vi "approach.vi"(8 "error in (no error)":errorcluster, 11 "Input":string="f") -> (0 "error out":errorcluster, 3 "Output":string="approached")   [LabVIEW 2014]
uses:
  <userlib>/Nanonis Prog Interface V5/Nanonis Prog Interface.lvlib
  <userlib>/SSL Library/SSL Lib.lvlib
panel:
  in  "Amplitude (V) (NaN=no change)":sgl=200.0
  in  "Frequency (Hz) (NaN=no change)":sgl=1000.0
  out "testing?":bool
  in  "STMStatus":T1 {"Size (m)"."Height" format="%.2p"; "Size (m)"."Width" format="%.2p"; "Current (A)" format="%#_6p"; "Z position (m)" format="%#_6p"; "Center coordinates (m)"."Yc" format="%.2p"; "Center coordinates (m)"."Xc" format="%.2p"}
  out "size(s)":i32=1
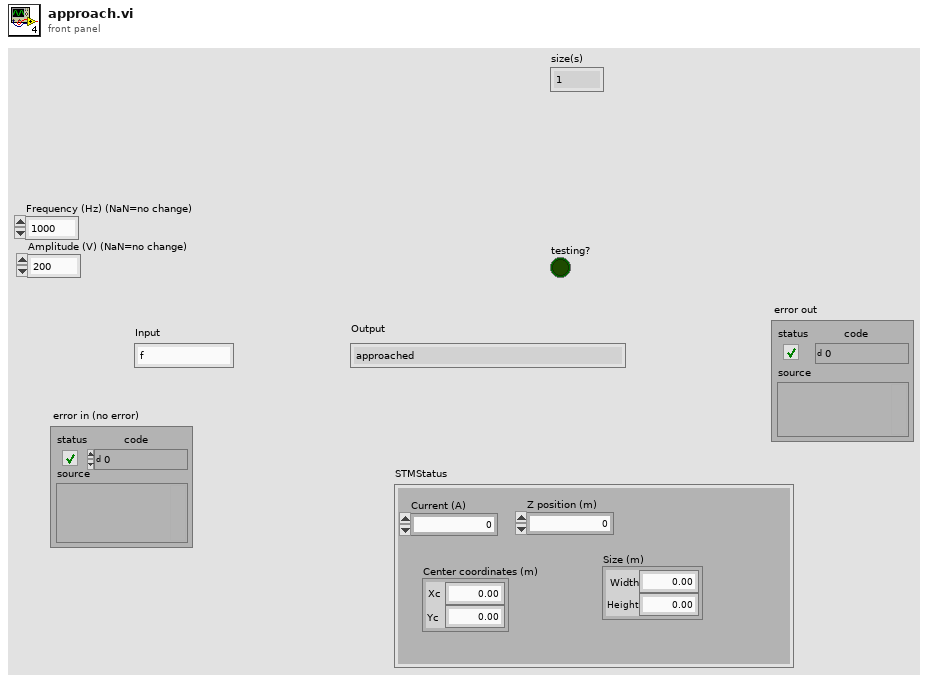
[diagram p1: front panel]
types:
  T1 = cluster{"Center coordinates (m)":cluster{"Xc":sgl, "Yc":sgl}, "Z position (m)":sgl, "Current (A)":sgl, "Size (m)":cluster{"Width":sgl, "Height":sgl}}
  T2 = enum8{"Group 1", "Group 2", "Group 3", "Group 4", "Group 5", "Group 6"}
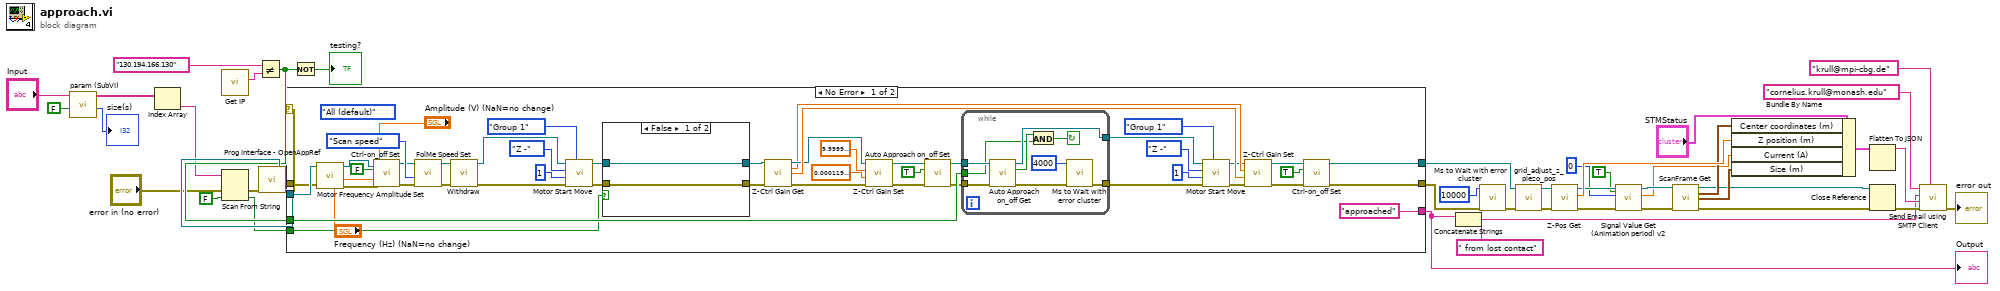
[diagram p0: block diagram]
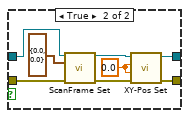
[diagram p2: hidden frame]
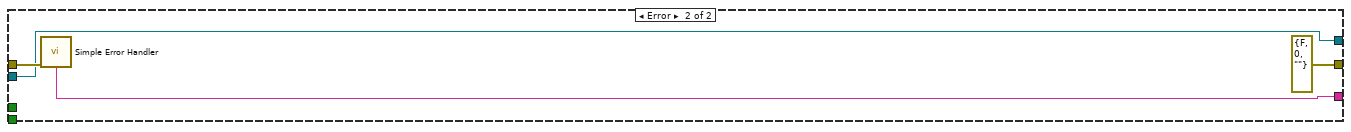
[diagram p3: hidden frame]
diagram:
  n1 = call <userlib>:"param (SubVI).vi"("Numeric"=FALSE, "Input"="Input") -> ("num"=→"size(s)":i32, "Array"=w18:string[])  [unwired: 7 in, 1 out]
  n2 = Index Array(array=w18) -> (element=w17:string)  [unwired: 1 in]
  n3 = call <userlib>:"Get IP.vi"() -> ("IP Address"=w22:string)  [unwired: 10 in, 1 out]
  n4 = Scan From String(input string=w17, error in="error in (no error)", default 1=FALSE) -> (error out=w15:errorcluster, output 1=w13:bool)  [unwired: 2 in, 2 out]
  n5 = Not Equal?(x="130.194.166.130" ("IP Address"), y=w22) -> (x != y?=w20:bool)
  n6 = call <userlib>:"Prog Interface - OpenAppRef.vi"("Error in (no error)"=w15) -> ("Error out"=w19:errorcluster, "Application reference"=w41:refnum<vi>)  [unwired: 5 in]
  n7 = case shown="No Error" w19 {
    tunnel: w41 -> [w50 w110]
    tunnel: w19 -> [w47 w113]
    tunnel: [w85 errorcluster {"status"=FALSE, "code"=0, "source"=""} ("error out")] -> w27
    tunnel: ["approached" ("initial string") w112] -> w10
    tunnel: [w84 w110] -> w7
    tunnel: w20 -> [w83 _]
    tunnel: w13 -> [w68 _]
    frame No Error {
      (unwired) enum16{"All (default)", "X", "Y", "Z"}."All (default)" ("Axis (All)")
      n8 = call <userlib>:"Motor Frequency Amplitude Set.vi"("Error in (no error)"=w47, "Amplitude (V) (NaN=no change)"="Amplitude (V) (NaN=no change)", "Frequency (Hz) (NaN=no change)"="Frequency (Hz) (NaN=no change)", "Application ref in"=w50) -> ("Error out"=w48:errorcluster, "Application ref out"=w49:refnum<vi>)  [unwired: 6 in]
      n9 = call <userlib>:"Ctrl-on_off Set.vi"("error in (no error)"=w48, "Z Controller ON/OFF"=FALSE, "Application ref in"=w49) -> ("error out"=w58:errorcluster, "Application ref out"=w44:refnum<vi>)  [unwired: 7 in]
      n10 = call <userlib>:"FolMe Speed Set.vi"("error in (no error)"=w58, "Speed Setting (Custom)"=enum32{"Scan speed", "Custom speed"}."Scan speed", "Application ref in"=w44) -> ("error out"=w88:errorcluster, "Application ref out"=w89:refnum<vi>)  [unwired: 5 in]
      n11 = call <userlib>:"Withdraw.vi"("Error in (no error)"=w88, "Application ref in"=w89) -> ("Error out"=w66:errorcluster, "Application ref out"=w67:refnum<vi>)  [unwired: 8 in]
      n12 = call <userlib>:"Motor Start Move.vi"("Group"=T2."Group 1", "Error in (no error)"=w66, "Number of steps"=u16 1, "Direction"=enum16{"X +", "X -", "Y +", "Y -", "Z +", "Z -"}."Z -", "Application ref in"=w67) -> ("Error out"=w64:errorcluster, "Application ref out"=w65:refnum<vi>)  [unwired: 4 in]
      n13 = case shown="False" w68 {
        tunnel: w65 -> [w91 w100]
        tunnel: w64 -> [w92 w99]
        tunnel: [w91 w94] -> w60
        tunnel: [w92 w93] -> w59
        frame False {
        }
        frame True {
          w95 = sgl 0.0 ("X (m)")
          n14 = call <userlib>:"ScanFrame Set.vi"("Application ref in"=w100, "Center coordinates (m)"=cluster{"Xc":sgl, "Yc":sgl} {"Xc"=0.0, "Yc"=0.0}, "error in (no error)"=w99) -> ("Application ref out"=w96:refnum<vi>, "error out"=w97:errorcluster)  [unwired: 11 in]
          n15 = call <userlib>:"XY-Pos Set.vi"("error in (no error)"=w97, "Y (m)"=w95, "X (m)"=w95, "Application ref in"=w96) -> ("error out"=w93:errorcluster, "Application ref out"=w94:refnum<vi>)  [unwired: 4 in]
        }
      }
      n16 = call <userlib>:"Z-Ctrl Gain Get.vi"("Application ref in"=w60, "error in (no error)"=w59) -> ("Application ref out"=w79:refnum<vi>, "P-gain"=w77:sgl, "Time constant (s)"=w82:sgl, "error out"=w74:errorcluster)  [unwired: 9 in, 1 out]
      n17 = call <userlib>:"Z-Ctrl Gain Set.vi"("error in (no error)"=w74, "Time constant (s)"=sgl 0.00012, "P-gain"=sgl 1e-11, "Application ref in"=w79) -> ("error out"=w73:errorcluster, "Application ref out"=w78:refnum<vi>)  [unwired: 5 in]
      n18 = call <userlib>:"Auto Approach on_off Set.vi"("Error in (no error)"=w73, "Auto approach start/stop (F)"=TRUE, "Application ref in"=w78) -> ("Error out"=w72:errorcluster, "Application ref out"=w75:refnum<vi>)  [unwired: 5 in]
      n19 = while {
        tunnel: w75 -> [w107]
        tunnel: [w106] -> w55
        tunnel: w72 -> [w105]
        tunnel: [w104] -> w57
        tunnel: w83 -> [w101]
        stop <- w102 continue-if-true
        n20 = call <userlib>:"Auto Approach on_off Get.vi"("Error in (no error)"=w105, "Application ref in"=w107) -> ("Error out"=w108:errorcluster, "Auto approach on/off status"=w103:bool, "Application ref out"=w106:refnum<vi>)  [unwired: 5 in]
        n21 = And(x=w103, y=w101) -> (x .and. y?=w102:bool)
        n22 = call <userlib>:"Ms to Wait with error cluster.vi"("error in (no error)"=w108, "milliseconds to wait"=u32 4000) -> ("error out"=w104:errorcluster)  [unwired: 4 in, 1 out]
      }
      n23 = call <userlib>:"Motor Start Move.vi"("Group"=T2."Group 1", "Error in (no error)"=w57, "Number of steps"=u16 1, "Direction"=enum16{"X +", "X -", "Y +", "Y -", "Z +", "Z -"}."Z -", "Application ref in"=w55) -> ("Error out"=w56:errorcluster, "Application ref out"=w54:refnum<vi>)  [unwired: 4 in]
      n24 = call <userlib>:"Z-Ctrl Gain Set.vi"("error in (no error)"=w56, "Time constant (s)"=w82, "P-gain"=w77, "Application ref in"=w54) -> ("error out"=w69:errorcluster, "Application ref out"=w71:refnum<vi>)  [unwired: 5 in]
      n25 = call <userlib>:"Ctrl-on_off Set.vi"("error in (no error)"=w69, "Z Controller ON/OFF"=TRUE, "Application ref in"=w71) -> ("error out"=w85:errorcluster, "Application ref out"=w84:refnum<vi>)  [unwired: 7 in]
    }
    frame Error {
      n26 = call <vilib>:"Simple Error Handler.vi"("error in (no error)"=w113) -> ("message"=w112:string)  [unwired: 4 in, 4 out]
    }
  }
  "Output" <- w10
  n27 = Not(x=w20) -> (.not. x?=→"testing?":bool)
  n28 = Concatenate Strings(w10, " from lost contact" ("string")) -> (w2:string)
  n29 = call <userlib>:"Ms to Wait with error cluster.vi"("error in (no error)"=w27, "milliseconds to wait"=u32 10000) -> ("error out"=w4:errorcluster)  [unwired: 4 in, 1 out]
  n30 = call "grid_adjust_z_piezo_pos.vi"("Error in (no error)"=w4, "Application ref in"=w7) -> ("Error out"=w6:errorcluster, "Application ref out"=w5:refnum<vi>)  [unwired: 8 in]
  n31 = call <userlib>:"Z-Pos Get.vi"("error in (no error)"=w6, "Application ref in"=w5) -> ("error out"=w31:errorcluster, "Z position (m)"=w37:sgl, "Application ref out"=w34:refnum<vi>)  [unwired: 7 in]
  n32 = call <userlib>:"Signal Value Get (Animation period) v2.vi"("Wait for newest data (F=False)"=TRUE, "error in (no error)"=w31, "Signal index (0-79)"=i8 0, "Application ref in"=w34) -> ("error out"=w32:errorcluster, "Signal value"=w29:sgl, "Application ref out"=w33:refnum<vi>)  [unwired: 4 in]
  n33 = call <userlib>:"ScanFrame Get.vi"("Application ref in"=w33, "error in (no error)"=w32) -> ("Application ref out"=w25:refnum<vi>, "Center coordinates (m)"=w36:cluster{"Xc":sgl, "Yc":sgl}, "Size (m)"=w35:cluster{"Width":sgl, "Height":sgl}, "error out"=w24:errorcluster)  [unwired: 9 in, 1 out]
  n34 = Bundle By Name(cluster="STMStatus", "Center coordinates (m)"=w36, "Z position (m)"=w37, "Current (A)"=w29, "Size (m)"=w35) -> (w38:T1)
  n35 = Flatten To JSON(anything=w38) -> (JSON string=w11:string)  [unwired: 2 in, 1 out]
  n36 = Close Reference(reference=w25, error in (no error)=w24) -> (error out=w9:errorcluster)
  n37 = call "Send Email using SMTP Client.vi"("CC"="krull@mpi-cbg.de", "error in (no error)"=w9, "Message"=w11, "Subject"=w2, "To:"="cornelius.krull@monash.edu" ("Recipients")) -> ("error out"=→"error out":errorcluster)  [unwired: 6 in]
